vi "Parallel Event Struct.vi"() -> (0 "References":T1)   [LabVIEW 2019]
uses:
  PV Info.ctl
  CaLab.lvlib
panel:
  out "Status":bool=TRUE
  out "PV Info":T2={"Name"="", "Elements"=0, "Values (string)"=[""], "Values (number)"=[0.0], "Status (string)"="", "Status (number)"=0, "Severity (string)"="", "Severity (number)"=0, "Timestamp (string)"=" ", "Timestamp (number)"=0, "Field Names"=[], "Field Values"=[], "Error"={"status"=FALSE, "code"=0, "source"=""}}
  in  "Number Of Updates":i32
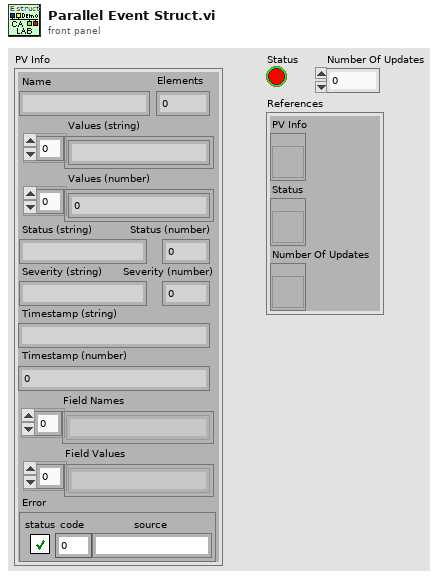
[diagram p1: front panel]
types:
  T1 = cluster{"PV Info":refnum<vi>, "Status":refnum<vi>, "Number Of Updates":refnum<vi>}
  T2 = typedef "CaLab.lvlib/PV Info.ctl" = cluster{"Name":string, "Elements":i32, "Values (string)":string[], "Values (number)":dbl[], "Status (string)":string, "Status (number)":i16, "Severity (string)":string, "Severity (number)":i16, "Timestamp (string)":string, "Timestamp (number)":i32, "Field Names":string[], "Field Values":string[], "Error":errorcluster}
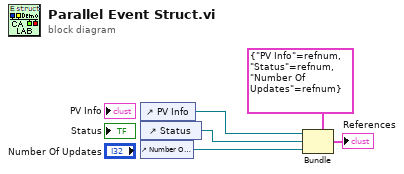
[diagram p0: block diagram]
diagram:
  n1 = control-ref of="PV Info"() -> (w5:refnum<vi>)
  n2 = control-ref of="Status"() -> (w4:refnum<vi>)
  n3 = control-ref of="Number Of Updates"() -> (w3:refnum<vi>)
  n4 = Bundle(cluster=T1 {"PV Info"=refnum, "Status"=refnum, "Number Of Updates"=refnum}, "PV Info"=w5, "Status"=w4, "Number Of Updates"=w3) -> (→"References":T1)
